vi "WriteFIFOConfig_HH.vi"(1 "error in (no error)":errorcluster) -> (0 "error out":errorcluster)   [LabVIEW 2009]
uses:
  SPCConfiguration.ctt
  FIFOSettings.ctt
  <vilib>/Utility/config.llb/NI_LVConfig.lvlib
panel:
  out "FIFO Settings":T1={"Measurement"={"Binning (ms)"=4719.0, "External Trigger Condition"=14979, "Stop Condition:"=0, "Stop Count"=0.0, "Buffer Size (Photons)"=30000, "No of Channels"=1, "Ext Latch Delay"=0}, "ADC"={"Binning (HH)"=0, "Dither Range"=0, "Count Increment"=0, "Mode"=1}, "SYNC"={"SYNC ZC Level (mV)"=-49.889763, "SYNC Freq Divider"=1, "SYNC Holdoff (ps)"=4.0, "SYNC Threshold (mV)"=-19.607843}, "TAC"={"TAC Range (ns)"=50.0, "TAC Gain"=0, "TAC Offset (%)"=0.0, "TAC Limit Low (%)"=0.0, "TAC Limit High (%)"=100.0}, "Ch 2"={"Ch2 ZC Level (mV)"=-43.137257, "Ch2 Holdoff (ps)"=67.76471, "Ch2 Threshold (mV)"=-49.889763}, "Ch 3"={"Ch3 ZC Level (mV)"=0.0, "Ch3 Holdoff (ps)"=4.0, "Ch3 Threshold (mV)"=200.0}, "Ch 4"={"Ch4 ZC Level (mV)"=0.0, "Ch4 Holdoff (ps)"=4.0, "Ch4 Threshold (mV)"=200.0}, "Ch1"={"Ch1 ZC Level (mV)"=0.0, "Ch1 Holdoff (ps)"=4.0, "Ch1 Threshold (mV)"=200.0}} {"Ch1"."Ch1 Threshold (mV)" min=0 max=1000 format="%.2f"; "Ch1"."Ch1 Holdoff (ps)" min=-99999 max=99999 format="%.2f"; "Ch1"."Ch1 ZC Level (mV)" min=0 max=40 format="%.2f"; "Ch 4"."Ch4 Threshold (mV)" min=0 max=1000 format="%.2f"; "Ch 4"."Ch4 Holdoff (ps)" min=-99999 max=99999 format="%.2f"; "Ch 4"."Ch4 ZC Level (mV)" min=0 max=40 format="%.2f"; "Ch 3"."Ch3 Threshold (mV)" min=0 max=1000 format="%.2f"; "Ch 3"."Ch3 Holdoff (ps)" min=-99999 max=99999 format="%.2f"; "Ch 3"."Ch3 ZC Level (mV)" min=0 max=40 format="%.2f"; "Ch 2"."Ch2 Threshold (mV)" min=-96 max=96 format="%.2f"; "Ch 2"."Ch2 Holdoff (ps)" min=4 max=80 format="%.2f"; "Ch 2"."Ch2 ZC Level (mV)" min=-500 max=80 format="%.2f"; "TAC"."TAC Limit High (%)" min=0 max=100 format="%.2f"; "TAC"."TAC Limit Low (%)" min=5 max=20 format="%.2f"; "TAC"."TAC Offset (%)" min=-96 max=96 format="%.2f"; "TAC"."TAC Gain" min=4 max=80; "TAC"."TAC Range (ns)" min=-500 max=80 format="%.2f"; "SYNC"."SYNC Threshold (mV)" min=5 max=20 format="%.2f"; "SYNC"."SYNC Holdoff (ps)" min=-96 max=96 format="%.2f"; "SYNC"."SYNC Freq Divider" items=["1", "2", "4", "8", "16"]; "SYNC"."SYNC ZC Level (mV)" min=-500 max=80 format="%.2f"; "ADC"."Mode" items=["T3"]; "ADC"."Binning (HH)" items=["1", "2", "4", "8", "16", "32", "64", "128", "256", "512", "1024"]; "ADC"."Count Increment" min=0 max=100; "ADC"."Dither Range" min=1 max=15 step=1; "Measurement"."Ext Latch Delay" min=0 max=255 step=1; "Measurement"."Stop Count" min=-500.0 max=-19.0 format="%.2f"; "Measurement"."Stop Condition:" items=["None", "Photon Count", "Time (s)"]; "Measurement"."External Trigger Condition" min=1 max=16 step=1; "Measurement"."No of Channels" max=14; "Measurement"."Binning (ms)" max=96 format="%.3f"}
  out "Storage Info (output)":cluster{"Store Data":bool, "Destination:":path}
  out "SPC Configuration":T2={"SPC Initialization File"=path "SPC Labview Drivers/Important/spcm.ini", "Module Number"=0, "Operation Mode"=0, "Trigger Channel"="0"}
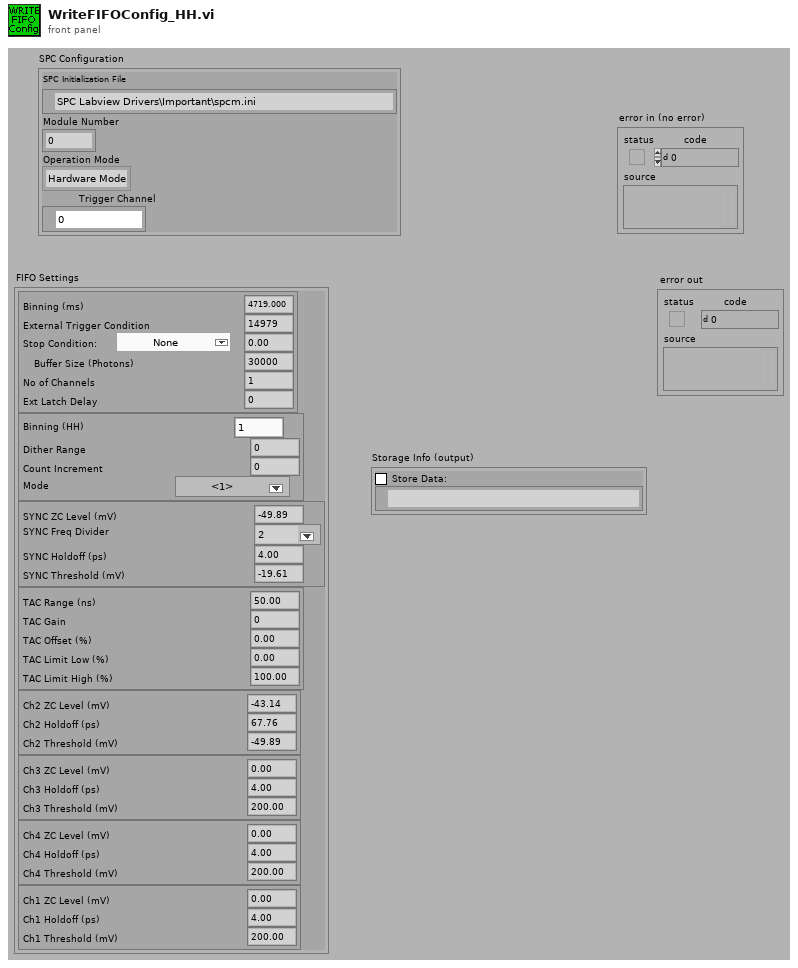
[diagram p1: front panel]
types:
  T1 = typedef "FIFOSettings.ctt" = cluster{"Measurement":cluster{"Binning (ms)":sgl, "External Trigger Condition":u16, "Stop Condition:":u16, "Stop Count":dbl, "Buffer Size (Photons)":u32, "No of Channels":u16, "Ext Latch Delay":i16}, "ADC":cluster{"Binning (HH)":i16, "Dither Range":i16, "Count Increment":i16, "Mode":u16}, "SYNC":cluster{"SYNC ZC Level (mV)":sgl, "SYNC Freq Divider":u16, "SYNC Holdoff (ps)":sgl, "SYNC Threshold (mV)":sgl}, "TAC":cluster{"TAC Range (ns)":sgl, "TAC Gain":i16, "TAC Offset (%)":sgl, "TAC Limit Low (%)":sgl, "TAC Limit High (%)":sgl}, "Ch 2":cluster{"Ch2 ZC Level (mV)":sgl, "Ch2 Holdoff (ps)":sgl, "Ch2 Threshold (mV)":sgl}, "Ch 3":cluster{"Ch3 ZC Level (mV)":sgl, "Ch3 Holdoff (ps)":sgl, "Ch3 Threshold (mV)":sgl}, "Ch 4":cluster{"Ch4 ZC Level (mV)":sgl, "Ch4 Holdoff (ps)":sgl, "Ch4 Threshold (mV)":sgl}, "Ch1":cluster{"Ch1 ZC Level (mV)":sgl, "Ch1 Holdoff (ps)":sgl, "Ch1 Threshold (mV)":sgl}}
  T2 = typedef "SPCConfiguration.ctt" = cluster{"SPC Initialization File":path, "Module Number":u16, "Operation Mode":u16, "Trigger Channel":tag}
  T3 = typedef "NI_LVConfig.lvlib/Config Data RefNum.ctl" = refnum<k1>
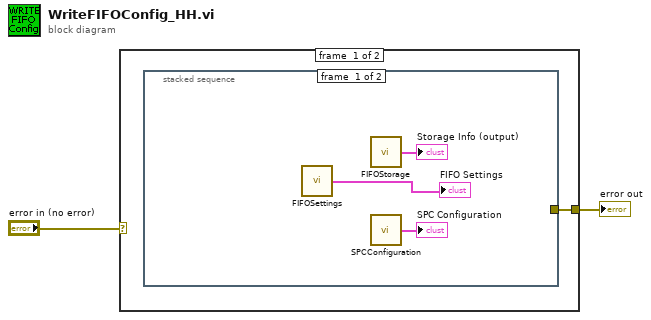
[diagram p0: block diagram]
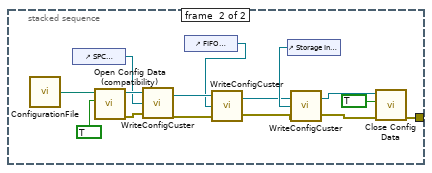
[diagram p2: hidden frame]
diagram:
  n1 = case shown="No Error" "error in (no error)" {
    selector: "error in (no error)" -> [_ w22]
    tunnel: [w3 w22] -> w2
    frame #0 {
      n2 = stacked-sequence {
        tunnel: [_ w20] -> w3
        frame #0 {
          n3 = call "FIFOSettings.vi"() -> ("FIFO Settings(out)"=→"FIFO Settings":T1)  [unwired: 2 in]
          n4 = call "FIFOStorage.vi"() -> ("Storage Info (output)"=→"Storage Info (output)":cluster{"Store Data":bool, "Destination:":path})  [unwired: 2 in]
          n5 = call "SPCConfiguration.vi"() -> ("SPC Configuration (output)"=→"SPC Configuration":T2)  [unwired: 2 in]
        }
        frame #1 {
          n6 = call "ConfigurationFile.vi"() -> ("Configuration File (output)"=w8:path)  [unwired: 2 in]
          n7 = control-ref of="SPC Configuration"() -> (w16:refnum<vi>)
          n8 = call <vilib>:"Open Config Data (compatibility).vi"("create file if necessary (T)"=TRUE ("create file if necessary? (T)"), "configuration file path"=w8) -> ("error out"=w17:errorcluster, "refnum"=w18:T3)  [unwired: 7 in, 1 out]
          n9 = call "WriteConfigCuster.vi"("error in (no error)"=w17, "Ctrl Reference"=w16, "ConfigFile (input)"=w18) -> ("error out"=w9:errorcluster, "ConfigFile (output)"=w12:T3)
          n10 = control-ref of="FIFO Settings"() -> (w7:refnum<vi>)
          n11 = call "WriteConfigCuster.vi"("error in (no error)"=w9, "Ctrl Reference"=w7, "ConfigFile (input)"=w12) -> ("error out"=w10:errorcluster, "ConfigFile (output)"=w11:T3)
          n12 = control-ref of="Storage Info (output)"() -> (w15:refnum<vi>)
          n13 = call "WriteConfigCuster.vi"("error in (no error)"=w10, "Ctrl Reference"=w15, "ConfigFile (input)"=w11) -> ("error out"=w13:errorcluster, "ConfigFile (output)"=w14:T3)
          n14 = call "Close Config Data.vi"("error in (no error)"=w13, "write configuration file? (T)"=TRUE ("write configuration file? (F)"), "refnum"=w14) -> ("error out"=w20:errorcluster)  [unwired: 8 in]
        }
      }
    }
    frame #1 {
    }
  }
  "error out" <- w2
